vi "Do Turn.vi"(9 "Teams In":refnum<class "Team.lvclass">[](array[class]), 10 "Round":u32, 11 "Map in":refnum<class "Map.lvclass">) -> (1 "Teams":refnum<class "Team.lvclass">[](array[class]), 3 "Map out":refnum<class "Map.lvclass">)   [LabVIEW 2020, in "SquareBattle.lvlib" / "Map.lvclass"]
uses:
  Map.lvclass
  Team/Team.lvclass
  e5ecc16e-3bff-46b9-858d-91a6d832ff84.vi
  82ce67f6-5fef-4b16-9808-9b19183b45dc.vi
  ab0dc01f-f0aa-44f7-a29f-68322b17ac23.vi
  <vilib>/Utility/High Resolution Relative Seconds.vi
panel:
  out "Collect":dbl
  out "Resolve":dbl
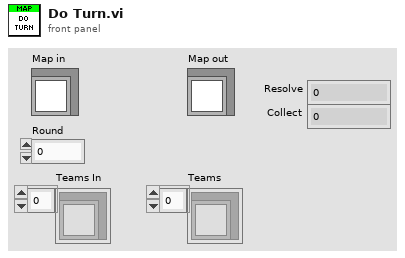
[diagram p1: front panel]
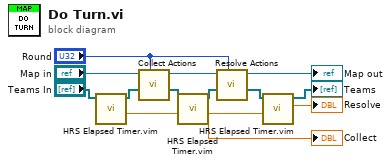
[diagram p0: block diagram]
diagram:
  n1 = call "HRS Elapsed Timer.vim"("Top In"="Teams In") -> ("HRS"=w4:dbl, "Top"=w9:refnum<class "Team.lvclass">[])  [unwired: 7 in, 2 out]
  n2 = call "Collect Actions.vi"("Round"="Round", "Teams In"=w9, "Map in"="Map in") -> ("Teams"=w8:refnum<class "Team.lvclass">[], "Map out"=w13:refnum<class "Map.lvclass">)  [unwired: 7 in]
  n3 = call "HRS Elapsed Timer.vim"("HRS In"=w4, "Top In"=w8) -> ("HRS"=w3:dbl, "Elapsed"=→"Collect":dbl, "Top"=w7:refnum<class "Team.lvclass">[])  [unwired: 6 in, 1 out]
  n4 = call "Resolve Actions.vi"("Round"="Round", "Teams in"=w7, "Map in"=w13) -> ("Teams out"=w6:refnum<class "Team.lvclass">[], "Map out"=→"Map out":refnum<class "Map.lvclass">)  [unwired: 7 in]
  n5 = call "HRS Elapsed Timer.vim"("HRS In"=w3, "Top In"=w6) -> ("Elapsed"=→"Resolve":dbl, "Top"=→"Teams":refnum<class "Team.lvclass">[])  [unwired: 6 in, 2 out]
